vi "Lian_Lab07_III.vi"() -> ()   [LabVIEW 2020]
uses:
  <vilib>/DAQmx/read.llb/DAQmx Read (Counter DBL 1Chan 1Samp).vi
  <vilib>/DAQmx/create/channels.llb/DAQmx Create Channel (CI-Frequency).vi
  <vilib>/DAQmx/miscellaneous.llb/DAQmx Fill In Error Info.vi
panel:
  in  "Scale Mod":dbl=1.0
  out "Waveform Chart 2":dbl(graph)
  in  "?":bool
  in  "Loop Delay (ms)":u32
  in  "Counter Channel":tag
  out "Waveform Chart 1":dbl(graph)
  # "Patr II."
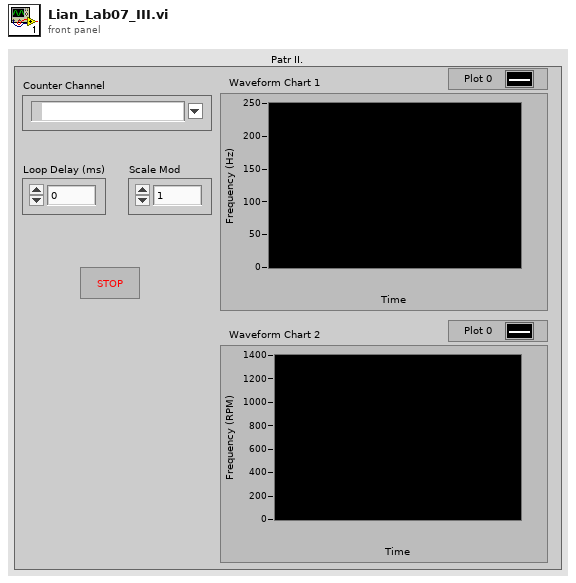
[diagram p1: front panel]
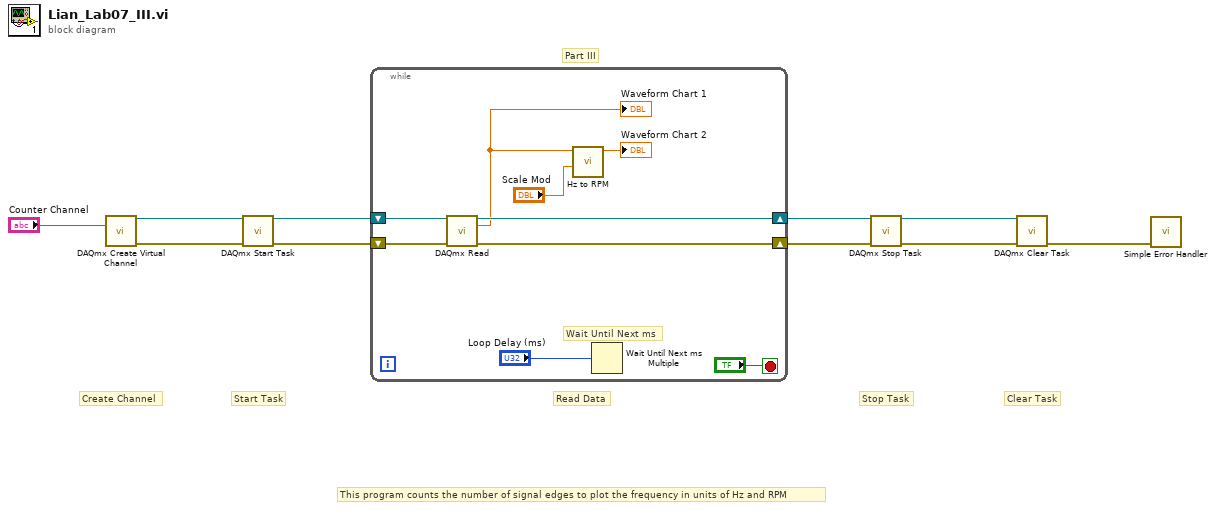
[diagram p0: block diagram]
diagram:
  # "This program counts the number of signal edges to plot the frequency in units of Hz and RPM"
  # "Read Data"
  # "Clear Task"
  # "Stop Task"
  # "Start Task"
  # "Create Channel"
  # "Part III"
  n1 = call-poly <vilib>:"DAQmx Create Virtual Channel.vi"("counter"="Counter Channel") -> ("task out"=w2:refnum<k21>, "error out"=w1:errorcluster)  [unwired: 13 in]
  n2 = call <vilib>:"DAQmx Start Task.vi"("task/channels in"=w2, "error in"=w1) -> ("task out"=w9:refnum<k21>, "error out"=w3:errorcluster)  [unwired: 12 in]
  n3 = while {
    shift-right: [w18] -> w8
    shift-left: w9 -> [w19]
    shift-right: [w17] -> w4
    shift-left: w3 -> [w16]
    stop <- "?" stop-if-true
    # "Wait Until Next ms"
    n4 = call-poly <vilib>:"DAQmx Read.vi"("task/channels in"=w19, "error in"=w16) -> ("task out"=w18:refnum<k21>, "data"=w12:dbl, "error out"=w17:errorcluster)  [unwired: 11 in]
    "Waveform Chart 1" <- w12
    n5 = call "Hz to RPM.vi"("Scale Mod"="Scale Mod", "Hz"=w12) -> ("RPM"=→"Waveform Chart 2":dbl)  [unwired: 9 in]
    n6 = Wait Until Next ms Multiple(millisecond multiple="Loop Delay (ms)") -> ()  [unwired: 1 out]
  }
  n7 = call <vilib>:"DAQmx Stop Task.vi"("task/channels in"=w8, "error in"=w4) -> ("task out"=w7:refnum<k21>, "error out"=w5:errorcluster)  [unwired: 12 in]
  n8 = call <vilib>:"DAQmx Clear Task.vi"("task in"=w7, "error in"=w5) -> ("error out"=w6:errorcluster)  [unwired: 13 in]
  n9 = call <vilib>:"Simple Error Handler.vi"("error in (no error)"=w6) -> ()  [unwired: 4 in, 5 out]
